vi "Teleop.vi"(10 "Match Info":T1={"Autonomous Elapsed Seconds"=0.0, "TeleOp Elapsed Seconds"=0.0, "Disabled Elapsed Seconds"=0.0, "Visited Autonomous"=FALSE, "Visited TeleOp"=FALSE, "Visited Disabled"=FALSE, "Autonomous Settings"={"Autonomous Style"=enum."Independent", "VI Refnum"=refnum}}, 11 "Call Context":T2) -> ()   [LabVIEW 2019]
doc: "This VI is called for each TeleOp packet received from the DS where the robot is not disabled. It is often used to read from the joysticks and update I/O or to update setpoints for timed control loops. It should complete and return within 20 milliseconds or it may miss DS packets."
uses:
  <vilib>/Rock Robotics/WPI/DriverStation/WPI_DriverStationDerivedRobotMode.ctl
  <vilib>/Rock Robotics/WPI/DriverStation/WPI_DriverStationMatch Info.ctl
  <vilib>/Rock Robotics/WPI/Utilities/WPI_GetSetVariantRefNum.vi
  <vilib>/Rock Robotics/Network Tables/NT Write Boolean Array.vi
  <vilib>/Rock Robotics/Network Tables/NT Write Numeric Array.vi
  <vilib>/Rock Robotics/Network Tables/NT Read Boolean.vi
  <vilib>/Rock Robotics/Network Tables/NT Write Boolean.vi
  <vilib>/Rock Robotics/Network Tables/NT Write Number.vi
  <vilib>/Rock Robotics/Network Tables/NT Read Number.vi
  <vilib>/Rock Robotics/Network Tables/NT Write String.vi
panel:
  out "Sample Slider 0":dbl(slide) scale=0.0..5.0
  out "Sample Boolean 1":bool
  out "Sample Boolean 0":bool
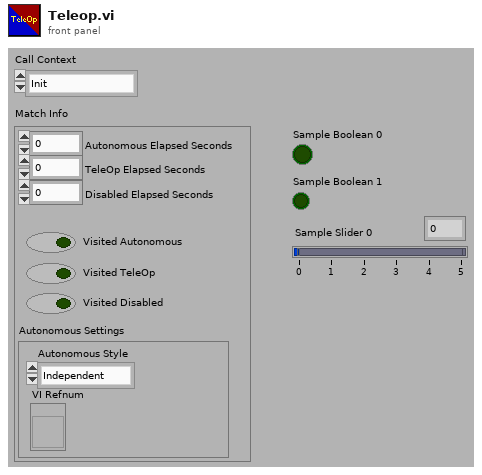
[diagram p1: front panel]
types:
  T1 = typedef "WPI_DriverStationMatch Info.ctl" = cluster{"Autonomous Elapsed Seconds":dbl, "TeleOp Elapsed Seconds":dbl, "Disabled Elapsed Seconds":dbl, "Visited Autonomous":bool, "Visited TeleOp":bool, "Visited Disabled":bool, "Autonomous Settings":cluster{"Autonomous Style":enum16{"Iterative", "Independent"}, "VI Refnum":refnum<vi>}}
  T2 = typedef "WPI_DriverStationDerivedRobotMode.ctl" = enum16{"Init", "Execute", "Stop"}
  T3 = typedef "WPI_JoystickDevRef.ctl" = cluster{"Device":T4}
  T4 = typedef "WPI_JoystickDeviceEnum.ctl" = enum16{"USB 0", "USB 1", "USB 2", "USB 3", "USB 4", "USB 5"}
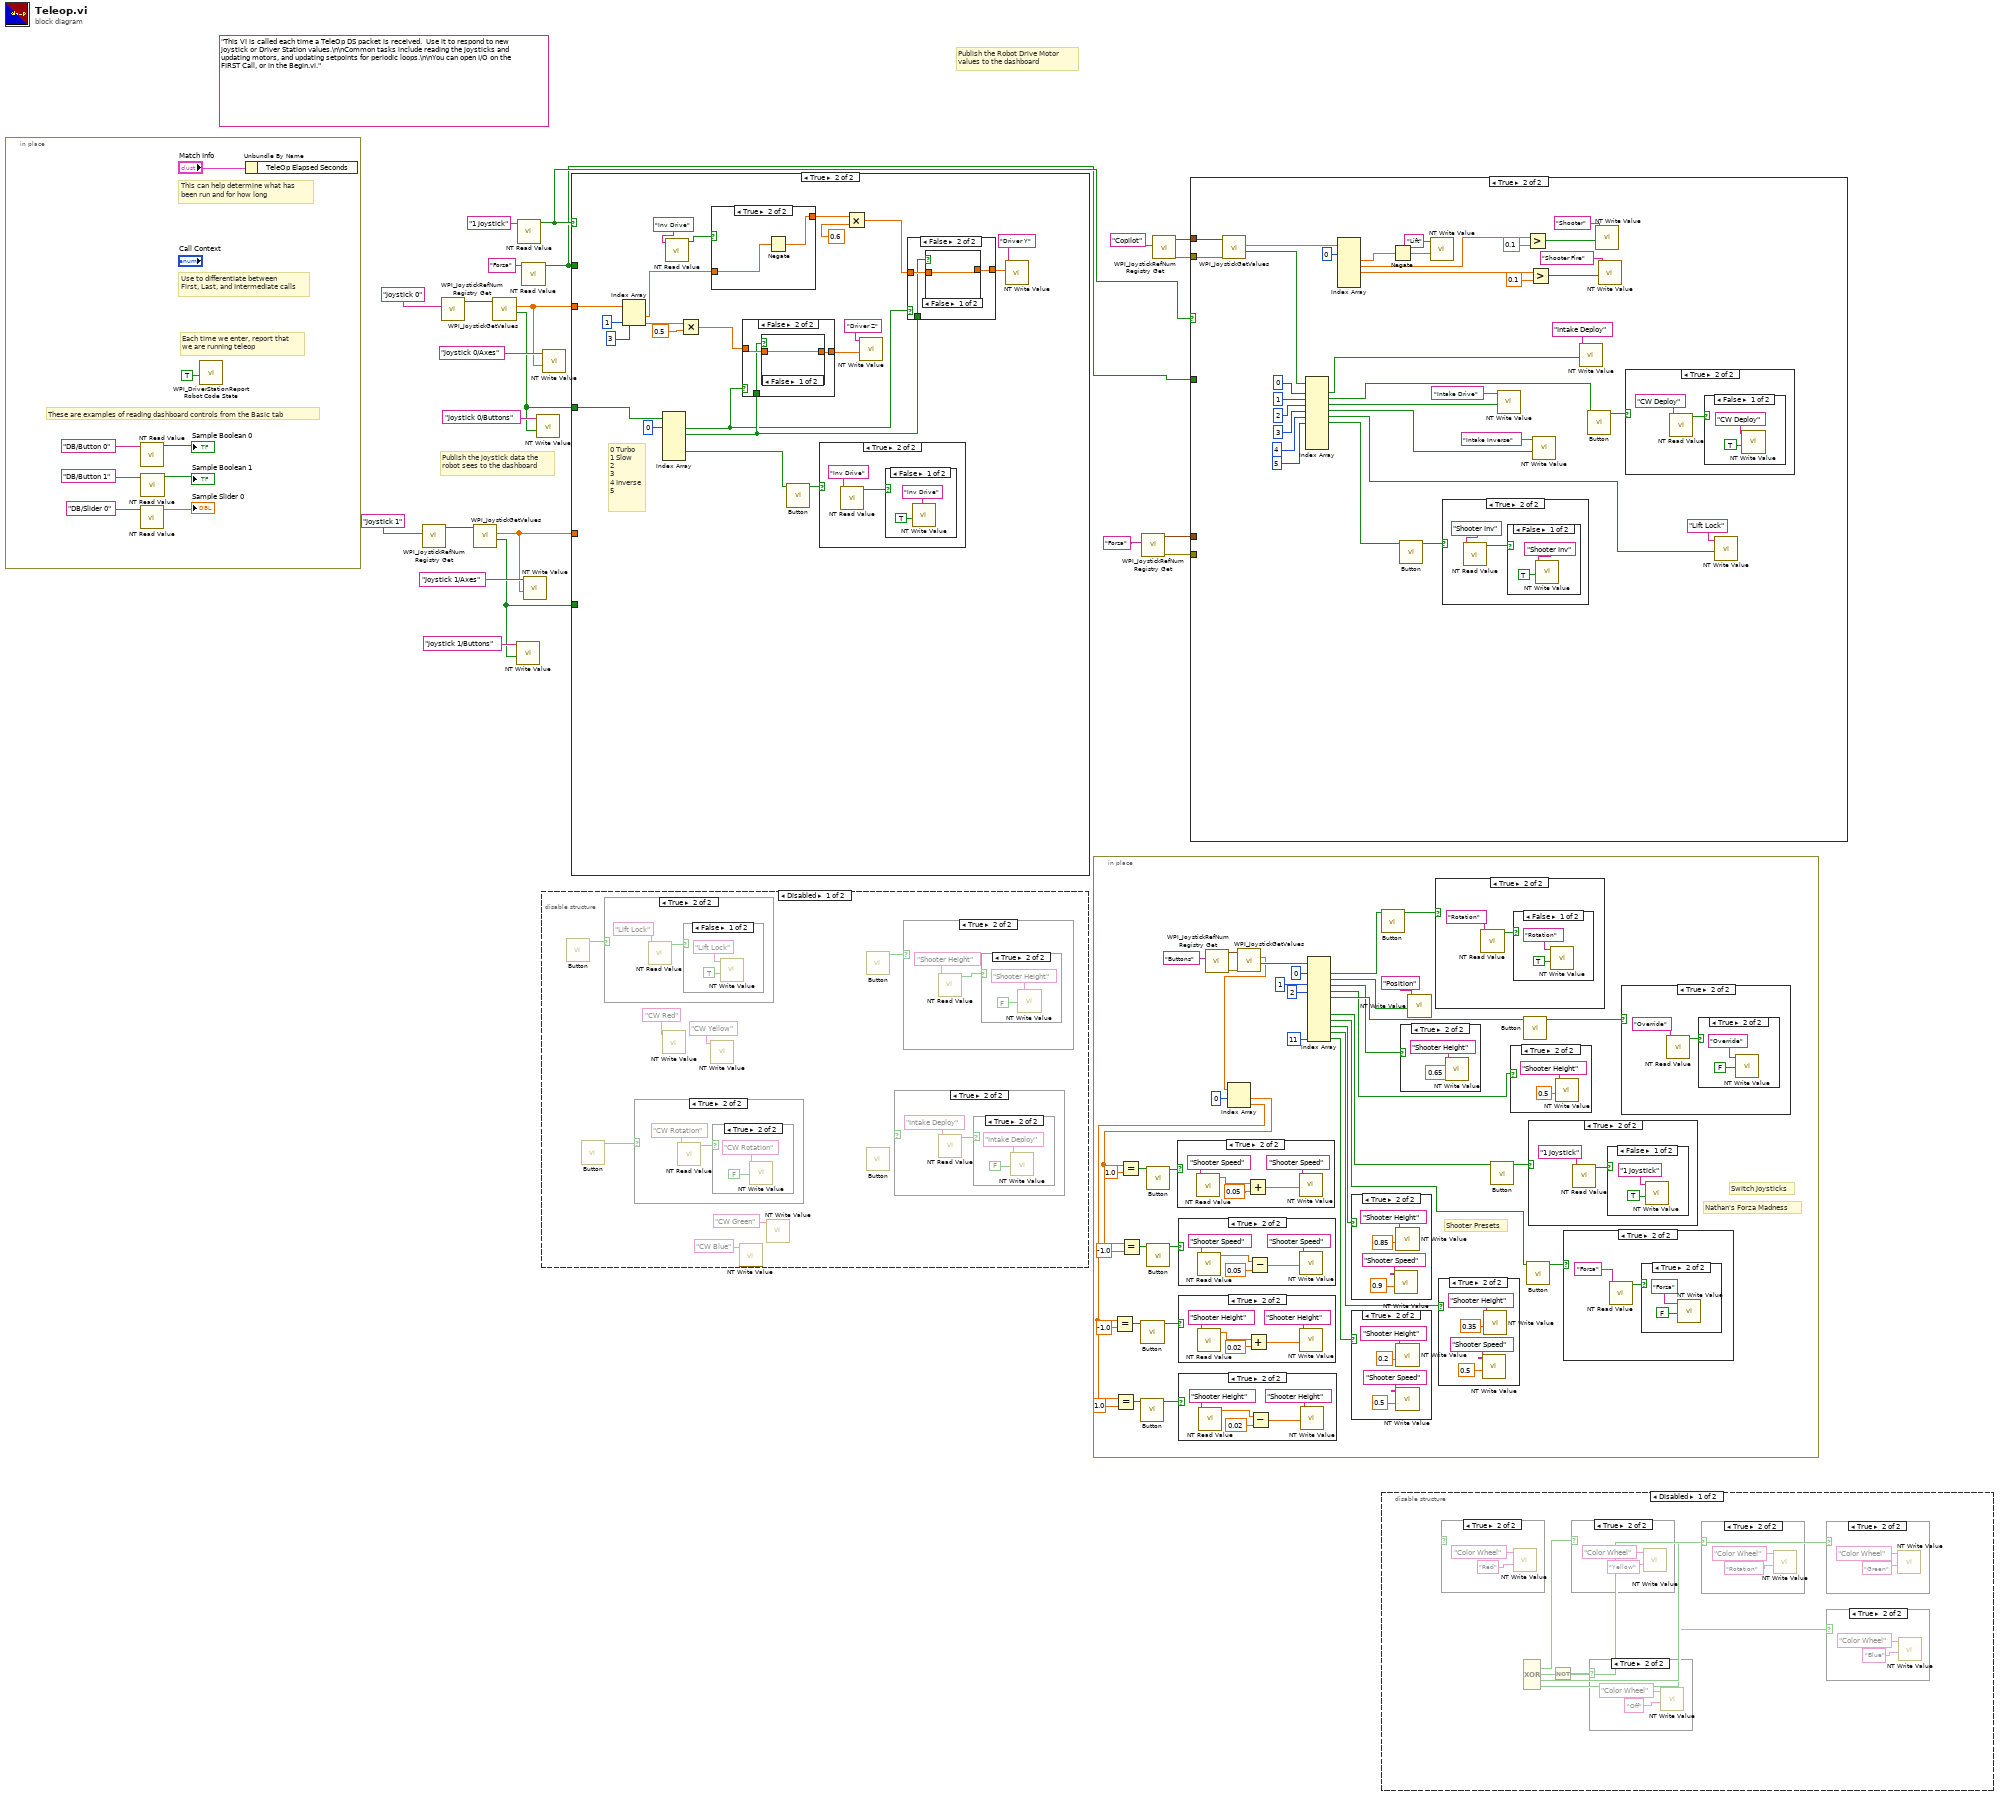
[diagram p0: block diagram]
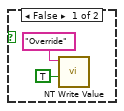
[diagram p9: hidden frame]
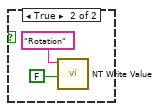
[diagram p11: hidden frame]
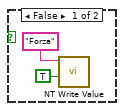
[diagram p14: hidden frame]
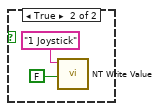
[diagram p16: hidden frame]
diagram:
  (unwired) "This VI is called each time a TeleOp DS packet is received.  Use it to respond to new joystick or Driver Station values.\n\nCommon tasks include reading the joysticks and updating motors, and updating setpoints for periodic loops.\n\nYou can open I/O on the FIRST Call, or in the Begin.vi."
  # "Publish the Robot Drive Motor\nvalues to the dashboard"
  # "Publish the joystick data the\nrobot sees to the dashboard"
  n1 = in-place {
    # "These are examples of reading dashboard controls from the Basic tab"
    # "Each time we enter, report that\nwe are running teleop"
    # "Use to differentiate between\nFirst, Last, and Intermediate calls"
    # "This can help determine what has\nbeen run and for how long"
    n2 = call-poly <vilib>:"NT Read Value.vi"("Name"="DB/Button 0" ("refnum name")) -> ("Boolean"=→"Sample Boolean 0":bool)  [unwired: 9 in, 1 out]
    n3 = call-poly <vilib>:"NT Read Value.vi"("Name"="DB/Slider 0" ("refnum name")) -> ("Numeric"=→"Sample Slider 0":dbl)  [unwired: 9 in, 1 out]
    n4 = call-poly <vilib>:"NT Read Value.vi"("Name"="DB/Button 1" ("refnum name")) -> ("Boolean"=→"Sample Boolean 1":bool)  [unwired: 9 in, 1 out]
    n5 = call <vilib>:"WPI_DriverStationReport Robot Code State.vi"("TeleOp"=TRUE ("Autonomous")) -> ()  [unwired: 10 in, 1 out]
    n6 = Unbundle By Name("Match Info") -> ()  [unwired: 1 out]
  }
  n7 = call <vilib>:"WPI_JoystickRefNum Registry Get.vi"("refnum name"="Joystick 1") -> ("JoystickDevRef"=w11:T3)  [unwired: 1 in, 9 out]
  n8 = call <vilib>:"WPI_JoystickRefNum Registry Get.vi"("refnum name"="Joystick 0") -> ("JoystickDevRef"=w21:T3)  [unwired: 1 in, 9 out]
  n9 = call <vilib>:"WPI_JoystickGetValues.vi"("JoystickDevRef"=w11) -> ("Buttons"=w7:bool[], "Axes"=w8:dbl[])  [unwired: 6 in, 3 out]
  n10 = call <vilib>:"WPI_JoystickGetValues.vi"("JoystickDevRef"=w21) -> ("Buttons"=w17:bool[], "Axes"=w18:dbl[])  [unwired: 6 in, 3 out]
  n11 = call-poly <vilib>:"NT Write Value.vi"("Boolean Array"=w7, "Name"="Joystick 1/Buttons") -> ()  [unwired: 9 in, 1 out]
  n12 = call-poly <vilib>:"NT Read Value.vi"("Name"="1 Joystick") -> ("Boolean"=w2:bool)  [unwired: 9 in, 1 out]
  n13 = call-poly <vilib>:"NT Read Value.vi"("Name"="Forza") -> ("Boolean"=w1:bool)  [unwired: 9 in, 1 out]
  n14 = call-poly <vilib>:"NT Write Value.vi"("Numeric Array"=w8, "Name"="Joystick 1/Axes") -> ()  [unwired: 9 in, 1 out]
  n15 = call-poly <vilib>:"NT Write Value.vi"("Boolean Array"=w17, "Name"="Joystick 0/Buttons") -> ()  [unwired: 9 in, 1 out]
  n16 = disable-structure shown="Disabled" {
    frame Disabled {
      n17 = call "Button.vi"() -> ("Button Pressed?"=w36:bool)  [unwired: 11 in]
      n18 = call "Button.vi"() -> ("Button Pressed?"=w31:bool)  [unwired: 11 in]
      n19 = case shown="True" w36 {
        frame False {
        }
        frame True {
          n20 = call-poly <vilib>:"NT Read Value.vi"("Name"="Lift Lock") -> ("Boolean"=w45:bool)  [unwired: 9 in, 1 out]
          n21 = case shown="False" w45 {
            frame False {
              n22 = call-poly <vilib>:"NT Write Value.vi"("Boolean"=TRUE, "Name"="Lift Lock") -> ()  [unwired: 9 in, 1 out]
            }
            frame True {
              n23 = call-poly <vilib>:"NT Write Value.vi"("Boolean"=FALSE, "Name"="Lift Lock") -> ()  [unwired: 9 in, 1 out]
            }
          }
        }
      }
      n24 = case shown="True" w31 {
        frame False {
        }
        frame True {
          n25 = call-poly <vilib>:"NT Read Value.vi"("Name"="CW Rotation") -> ("Boolean"=w39:bool)  [unwired: 9 in, 1 out]
          n26 = case shown="True" w39 {
            frame False {
              n27 = call-poly <vilib>:"NT Write Value.vi"("Boolean"=TRUE, "Name"="CW Rotation") -> ()  [unwired: 9 in, 1 out]
            }
            frame True {
              n28 = call-poly <vilib>:"NT Write Value.vi"("Boolean"=FALSE, "Name"="CW Rotation") -> ()  [unwired: 9 in, 1 out]
            }
          }
        }
      }
      n29 = call-poly <vilib>:"NT Write Value.vi"("Name"="CW Red") -> ()  [unwired: 10 in, 1 out]
      n30 = call-poly <vilib>:"NT Write Value.vi"("Name"="CW Yellow") -> ()  [unwired: 10 in, 1 out]
      n31 = call-poly <vilib>:"NT Write Value.vi"("Name"="CW Blue") -> ()  [unwired: 10 in, 1 out]
      n32 = call-poly <vilib>:"NT Write Value.vi"("Name"="CW Green") -> ()  [unwired: 10 in, 1 out]
      n33 = call "Button.vi"() -> ("Button Pressed?"=w38:bool)  [unwired: 11 in]
      n34 = call "Button.vi"() -> ()  [unwired: 11 in, 1 out]
      n35 = case shown="True" w37 {
        frame False {
        }
        frame True {
          n36 = call-poly <vilib>:"NT Read Value.vi"("Name"="Intake Deploy") -> ("Boolean"=w51:bool)  [unwired: 9 in, 1 out]
          n37 = case shown="True" w51 {
            frame False {
              n38 = call-poly <vilib>:"NT Write Value.vi"("Boolean"=TRUE, "Name"="Intake Deploy") -> ()  [unwired: 9 in, 1 out]
            }
            frame True {
              n39 = call-poly <vilib>:"NT Write Value.vi"("Boolean"=FALSE, "Name"="Intake Deploy") -> ()  [unwired: 9 in, 1 out]
            }
          }
        }
      }
      n40 = case shown="True" w38 {
        frame False {
        }
        frame True {
          n41 = call-poly <vilib>:"NT Read Value.vi"("Name"="Shooter Height") -> ("Boolean"=w57:bool)  [unwired: 9 in, 1 out]
          n42 = case shown="True" w57 {
            frame False {
              n43 = call-poly <vilib>:"NT Write Value.vi"("Boolean"=TRUE, "Name"="Shooter Height") -> ()  [unwired: 9 in, 1 out]
            }
            frame True {
              n44 = call-poly <vilib>:"NT Write Value.vi"("Boolean"=FALSE, "Name"="Shooter Height") -> ()  [unwired: 9 in, 1 out]
            }
          }
        }
      }
    }
    frame Enabled {
    }
  }
  n45 = call-poly <vilib>:"NT Write Value.vi"("Numeric Array"=w18, "Name"="Joystick 0/Axes") -> ()  [unwired: 9 in, 1 out]
  n46 = case shown="True" w2 {
    tunnel: w18 -> [w67 w175]
    tunnel: w17 -> [w66 w174]
    tunnel: w8 -> [w65 _]
    tunnel: w7 -> [w64 _]
    tunnel: w1 -> [w63 _]
    frame False {
      n47 = case shown="False" w63 {
        tunnel: w67 -> [_ w101]
        tunnel: w66 -> [_ w100]
        tunnel: w65 -> [_ w99]
        tunnel: w64 -> [_ w97]
        frame True {
        }
        frame False {
          # "0 Fire Shooter\n1 Intake Run\n2 Intake Inverse\n3 Lift Lock\n4 Turbo\n5 CW Deploy"
          # "0 Rev Shooter\n1 Intake Deploy\n2\n3\n4 Inverse\n5 Slow"
          n48 = Index Array(array=w101, index=1) -> (element=w106:dbl)
          n49 = call-poly <vilib>:"NT Read Value.vi"("Name"="Inv Drive") -> ("Boolean"=w80:bool)  [unwired: 9 in, 1 out]
          n50 = Index Array(array=w97, index #1=0 ("index")) -> (element #1=w88:bool, element #2=w85:bool, element #3=w73:bool, element #4=w74:bool, element #5=w79:bool, element #6=w82:bool)  [unwired: 5 in]
          n51 = Index Array(array=w100, index #1=0) -> (element #1=w84:bool, element #2=w70:bool, element #3=w68:bool, element #5=w77:bool, element #6=w76:bool)  [unwired: 5 in, 1 out]
          n52 = Index Array(array=w99, index=1) -> (element=w96:dbl)
          n53 = case shown="True" w80 {
            tunnel: w106 -> [w141 w143]
            tunnel: [w141 w142] -> w105
            frame False {
            }
            frame True {
              n54 = Negate(x=w143) -> (-x=w142:dbl)
            }
          }
          n55 = case shown="True" w80 {
            tunnel: w96 -> [w138 w140]
            tunnel: [w138 w139] -> w91
            frame False {
            }
            frame True {
              n56 = Negate(x=w140) -> (-x=w139:dbl)
            }
          }
          n57 = call-poly <vilib>:"NT Write Value.vi"("Boolean"=w88, "Name"="Shooter Fire") -> ()  [unwired: 9 in, 1 out]
          n58 = call-poly <vilib>:"NT Write Value.vi"("Boolean"=w84, "Name"="Shooter") -> ()  [unwired: 9 in, 1 out]
          n59 = call-poly <vilib>:"NT Write Value.vi"("Boolean"=w85, "Name"="Intake Drive") -> ()  [unwired: 9 in, 1 out]
          n60 = call "Button.vi"("Button In"=w74) -> ("Button Pressed?"=w75:bool)  [unwired: 10 in]
          n61 = call-poly <vilib>:"NT Write Value.vi"("Boolean"=w73, "Name"="Intake Inverse") -> ()  [unwired: 9 in, 1 out]
          n62 = Multiply(x=w105, y=0.75) -> (x*y=w104:dbl)
          n63 = call-poly <vilib>:"NT Write Value.vi"("Boolean"=w70, "Name"="Intake Deploy") -> ()  [unwired: 9 in, 1 out]
          n64 = Multiply(x=w91, y=0.75) -> (x*y=w94:dbl)
          n65 = call "Button.vi"("Button In"=w82) -> ("Button Pressed?"=w83:bool)  [unwired: 10 in]
          n66 = call "Button.vi"("Button In"=w77) -> ("Button Pressed?"=w78:bool)  [unwired: 10 in]
          n67 = case shown="True" w75 {
            frame False {
            }
            frame True {
              n68 = call-poly <vilib>:"NT Read Value.vi"("Name"="Lift Lock") -> ("Boolean"=w110:bool)  [unwired: 9 in, 1 out]
              n69 = case shown="False" w110 {
                frame False {
                  n70 = call-poly <vilib>:"NT Write Value.vi"("Boolean"=TRUE, "Name"="Lift Lock") -> ()  [unwired: 9 in, 1 out]
                }
                frame True {
                  n71 = call-poly <vilib>:"NT Write Value.vi"("Boolean"=FALSE, "Name"="Lift Lock") -> ()  [unwired: 9 in, 1 out]
                }
              }
            }
          }
          n72 = case shown="True" w83 {
            frame False {
            }
            frame True {
              n73 = call-poly <vilib>:"NT Read Value.vi"("Name"="CW Deploy") -> ("Boolean"=w122:bool)  [unwired: 9 in, 1 out]
              n74 = case shown="False" w122 {
                frame False {
                  n75 = call-poly <vilib>:"NT Write Value.vi"("Boolean"=TRUE, "Name"="CW Deploy") -> ()  [unwired: 9 in, 1 out]
                }
                frame True {
                  n76 = call-poly <vilib>:"NT Write Value.vi"("Boolean"=FALSE, "Name"="CW Deploy") -> ()  [unwired: 9 in, 1 out]
                }
              }
            }
          }
          n77 = case shown="False" w79 {
            tunnel: w104 -> [w145 w149]
            tunnel: [w144 w148] -> w103
            tunnel: w76 -> [_ w147]
            frame True {
              n78 = Multiply(x=w145, y=1.33) -> (x*y=w144:dbl)
            }
            frame False {
              n79 = case shown="True" w147 {
                tunnel: w149 -> [w150 w152]
                tunnel: [w150 w151] -> w148
                frame False {
                }
                frame True {
                  n80 = Multiply(x=w152, y=0.66) -> (x*y=w151:dbl)
                }
              }
            }
          }
          n81 = case shown="False" w79 {
            tunnel: w94 -> [w129 w133]
            tunnel: [w128 w132] -> w93
            tunnel: w76 -> [_ w131]
            frame True {
              n82 = Multiply(x=w129, y=1.33) -> (x*y=w128:dbl)
            }
            frame False {
              n83 = case shown="True" w131 {
                tunnel: w133 -> [w134 w136]
                tunnel: [w134 w135] -> w132
                frame False {
                }
                frame True {
                  n84 = Multiply(x=w136, y=0.66) -> (x*y=w135:dbl)
                }
              }
            }
          }
          n85 = case shown="True" w78 {
            frame False {
            }
            frame True {
              n86 = call-poly <vilib>:"NT Read Value.vi"("Name"="Inv Drive") -> ("Boolean"=w116:bool)  [unwired: 9 in, 1 out]
              n87 = case shown="False" w116 {
                frame False {
                  n88 = call-poly <vilib>:"NT Write Value.vi"("Boolean"=TRUE, "Name"="Inv Drive") -> ()  [unwired: 9 in, 1 out]
                }
                frame True {
                  n89 = call-poly <vilib>:"NT Write Value.vi"("Boolean"=FALSE, "Name"="Inv Drive") -> ()  [unwired: 9 in, 1 out]
                }
              }
            }
          }
          n90 = call-poly <vilib>:"NT Write Value.vi"("Boolean"=w68, "Name"="Shooter Nerf") -> ()  [unwired: 9 in, 1 out]
          n91 = call-poly <vilib>:"NT Write Value.vi"("Numeric"=w103, "Name"="Driver Y") -> ()  [unwired: 9 in, 1 out]
          n92 = call-poly <vilib>:"NT Write Value.vi"("Numeric"=w93, "Name"="Driver Z") -> ()  [unwired: 9 in, 1 out]
        }
      }
    }
    frame True {
      # "0 Turbo\n1 Slow\n2\n3\n4 Inverse\n5"
      n93 = Index Array(array=w175, index #1=1, index #2=3) -> (element #1=w169:dbl, element #2=w164:dbl)
      n94 = Index Array(array=w174, index #1=0) -> (element #1=w158:bool, element #2=w159:bool, element #5=w156:bool)  [unwired: 5 in, 3 out]
      n95 = call-poly <vilib>:"NT Read Value.vi"("Name"="Inv Drive") -> ("Boolean"=w155:bool)  [unwired: 9 in, 1 out]
      n96 = Multiply(x=w164, y=0.5) -> (x*y=w165:dbl)
      n97 = case shown="True" w155 {
        tunnel: w169 -> [w192 w194]
        tunnel: [w192 w193] -> w168
        frame False {
        }
        frame True {
          n98 = Negate(x=w194) -> (-x=w193:dbl)
        }
      }
      n99 = case shown="False" w158 {
        tunnel: [w182 w186] -> w163
        tunnel: w165 -> [w183 w187]
        tunnel: w159 -> [_ w185]
        frame True {
          n100 = Multiply(x=w183, y=1.33) -> (x*y=w182:dbl)
        }
        frame False {
          n101 = case shown="False" w185 {
            tunnel: [w188 w190] -> w186
            tunnel: w187 -> [w188 w189]
            frame False {
            }
            frame True {
              n102 = Multiply(x=w189, y=0.66) -> (x*y=w190:dbl)
            }
          }
        }
      }
      n103 = call "Button.vi"("Button In"=w156) -> ("Button Pressed?"=w157:bool)  [unwired: 10 in]
      n104 = case shown="True" w157 {
        frame False {
        }
        frame True {
          n105 = call-poly <vilib>:"NT Read Value.vi"("Name"="Inv Drive") -> ("Boolean"=w176:bool)  [unwired: 9 in, 1 out]
          n106 = case shown="False" w176 {
            frame False {
              n107 = call-poly <vilib>:"NT Write Value.vi"("Boolean"=TRUE, "Name"="Inv Drive") -> ()  [unwired: 9 in, 1 out]
            }
            frame True {
              n108 = call-poly <vilib>:"NT Write Value.vi"("Boolean"=FALSE, "Name"="Inv Drive") -> ()  [unwired: 9 in, 1 out]
            }
          }
        }
      }
      n109 = Multiply(x=w168, y=0.6) -> (x*y=w167:dbl)
      n110 = call-poly <vilib>:"NT Write Value.vi"("Numeric"=w163, "Name"="Driver Z") -> ()  [unwired: 9 in, 1 out]
      n111 = case shown="False" w158 {
        tunnel: w167 -> [w196 w200]
        tunnel: [w195 w199] -> w161
        tunnel: w159 -> [_ w198]
        frame True {
          n112 = Multiply(x=w196, y=1.33) -> (x*y=w195:dbl)
        }
        frame False {
          n113 = case shown="False" w198 {
            tunnel: w200 -> [w201 w203]
            tunnel: [w201 w202] -> w199
            frame False {
            }
            frame True {
              n114 = Multiply(x=w203, y=0.66) -> (x*y=w202:dbl)
            }
          }
        }
      }
      n115 = call-poly <vilib>:"NT Write Value.vi"("Numeric"=w161, "Name"="Driver Y") -> ()  [unwired: 9 in, 1 out]
    }
  }
  n116 = in-place {
    # "Shooter Presets"
    # "Nathan's Forza Madness"
    # "Switch Joysticks"
    n117 = call <vilib>:"WPI_JoystickRefNum Registry Get.vi"("refnum name"="Buttons") -> ("error out"=w243:errorcluster, "JoystickDevRef"=w242:T3)  [unwired: 9 in]
    n118 = call <vilib>:"WPI_JoystickGetValues.vi"("error in (no error)"=w243, "JoystickDevRef"=w242) -> ("Buttons"=w240:bool[], "Axes"=w220:dbl[])  [unwired: 5 in, 3 out]
    n119 = Index Array(array=w220, index #1=0 ("index")) -> (element #1=w218:dbl, element #2=w213:dbl)  [unwired: 1 in]
    n120 = Equal?(x=w213, y=-1.0) -> (x = y?=w210:bool)
    n121 = Equal?(x=w213, y=1.0) -> (x = y?=w211:bool)
    n122 = Equal?(x=w218, y=1.0) -> (x = y?=w206:bool)
    n123 = Equal?(x=w218, y=-1.0) -> (x = y?=w208:bool)
    n124 = call "Button.vi"("Button In"=w211) -> ("Button Pressed?"=w212:bool)  [unwired: 10 in]
    n125 = call "Button.vi"("Button In"=w210) -> ("Button Pressed?"=w209:bool)  [unwired: 10 in]
    n126 = call "Button.vi"("Button In"=w206) -> ("Button Pressed?"=w205:bool)  [unwired: 10 in]
    n127 = call "Button.vi"("Button In"=w208) -> ("Button Pressed?"=w207:bool)  [unwired: 10 in]
    n128 = case shown="True" w205 {
      frame False {
      }
      frame True {
        n129 = call-poly <vilib>:"NT Read Value.vi"("Name"="Shooter Speed") -> ("Numeric"=w261:dbl)  [unwired: 9 in, 1 out]
        n130 = Add(x=w261, y=0.05) -> (x+y=w260:dbl)
        n131 = call-poly <vilib>:"NT Write Value.vi"("Numeric"=w260, "Name"="Shooter Speed") -> ()  [unwired: 9 in, 1 out]
      }
    }
    n132 = case shown="True" w207 {
      frame False {
      }
      frame True {
        n133 = call-poly <vilib>:"NT Read Value.vi"("Name"="Shooter Speed") -> ("Numeric"=w255:dbl)  [unwired: 9 in, 1 out]
        n134 = Subtract(x=w255, y=0.05) -> (x-y=w256:dbl)
        n135 = call-poly <vilib>:"NT Write Value.vi"("Numeric"=w256, "Name"="Shooter Speed") -> ()  [unwired: 9 in, 1 out]
      }
    }
    n136 = case shown="True" w209 {
      frame False {
      }
      frame True {
        n137 = call-poly <vilib>:"NT Read Value.vi"("Name"="Shooter Height") -> ("Numeric"=w251:dbl)  [unwired: 9 in, 1 out]
        n138 = Add(x=w251, y=0.02) -> (x+y=w250:dbl)
        n139 = call-poly <vilib>:"NT Write Value.vi"("Numeric"=w250, "Name"="Shooter Height") -> ()  [unwired: 9 in, 1 out]
      }
    }
    n140 = case shown="True" w212 {
      frame False {
      }
      frame True {
        n141 = call-poly <vilib>:"NT Read Value.vi"("Name"="Shooter Height") -> ("Numeric"=w245:dbl)  [unwired: 9 in, 1 out]
        n142 = Subtract(x=w245, y=0.02) -> (x-y=w246:dbl)
        n143 = call-poly <vilib>:"NT Write Value.vi"("Numeric"=w246, "Name"="Shooter Height") -> ()  [unwired: 9 in, 1 out]
      }
    }
    n144 = Index Array(array=w240, index #1=0 ("index"), index #2=1 ("index"), index #3=2 ("index"), index #12=11 ("index")) -> (element #1=w226:bool, element #2=w224:bool, element #3=w222:bool, element #4=w221:bool, element #5=w223:bool, element #8=w235:bool, element #9=w233:bool, element #10=w237:bool, element #11=w238:bool, element #12=w229:bool)  [unwired: 8 in, 2 out]
    n145 = case shown="True" w237 {
      frame False {
      }
      frame True {
        n146 = call-poly <vilib>:"NT Write Value.vi"("Numeric"=0.9, "Name"="Shooter Speed") -> ()  [unwired: 9 in, 1 out]
        n147 = call-poly <vilib>:"NT Write Value.vi"("Numeric"=0.85, "Name"="Shooter Height") -> ()  [unwired: 9 in, 1 out]
      }
    }
    n148 = case shown="True" w229 {
      frame False {
      }
      frame True {
        n149 = call-poly <vilib>:"NT Write Value.vi"("Numeric"=0.2, "Name"="Shooter Height") -> ()  [unwired: 9 in, 1 out]
        n150 = call-poly <vilib>:"NT Write Value.vi"("Numeric"=0.5, "Name"="Shooter Speed") -> ()  [unwired: 9 in, 1 out]
      }
    }
    n151 = call "Button.vi"("Button In"=w226) -> ("Button Pressed?"=w228:bool)  [unwired: 10 in]
    n152 = case shown="True" w222 {
      frame False {
      }
      frame True {
        n153 = call-poly <vilib>:"NT Write Value.vi"("Numeric"=0.65, "Name"="Shooter Height") -> ()  [unwired: 9 in, 1 out]
      }
    }
    n154 = call-poly <vilib>:"NT Write Value.vi"("Boolean"=w224, "Name"="Position") -> ()  [unwired: 9 in, 1 out]
    n155 = case shown="True" w228 {
      frame False {
      }
      frame True {
        n156 = call-poly <vilib>:"NT Read Value.vi"("Name"="Rotation") -> ("Boolean"=w274:bool)  [unwired: 9 in, 1 out]
        n157 = case shown="False" w274 {
          frame False {
            n158 = call-poly <vilib>:"NT Write Value.vi"("Boolean"=TRUE, "Name"="Rotation") -> ()  [unwired: 9 in, 1 out]
          }
          frame True {
            n159 = call-poly <vilib>:"NT Write Value.vi"("Boolean"=FALSE, "Name"="Rotation") -> ()  [unwired: 9 in, 1 out]
          }
        }
      }
    }
    n160 = case shown="True" w238 {
      frame False {
      }
      frame True {
        n161 = call-poly <vilib>:"NT Write Value.vi"("Numeric"=0.5, "Name"="Shooter Speed") -> ()  [unwired: 9 in, 1 out]
        n162 = call-poly <vilib>:"NT Write Value.vi"("Numeric"=0.35, "Name"="Shooter Height") -> ()  [unwired: 9 in, 1 out]
      }
    }
    n163 = call "Button.vi"("Button In"=w235) -> ("Button Pressed?"=w236:bool)  [unwired: 10 in]
    n164 = case shown="True" w221 {
      frame False {
      }
      frame True {
        n165 = call-poly <vilib>:"NT Write Value.vi"("Numeric"=0.5, "Name"="Shooter Height") -> ()  [unwired: 9 in, 1 out]
      }
    }
    n166 = call "Button.vi"("Button In"=w223) -> ("Button Pressed?"=w227:bool)  [unwired: 10 in]
    n167 = call "Button.vi"("Button In"=w233) -> ("Button Pressed?"=w234:bool)  [unwired: 10 in]
    n168 = case shown="True" w236 {
      frame False {
      }
      frame True {
        n169 = call-poly <vilib>:"NT Read Value.vi"("Name"="1 Joystick") -> ("Boolean"=w290:bool)  [unwired: 9 in, 1 out]
        n170 = case shown="False" w290 {
          frame False {
            n171 = call-poly <vilib>:"NT Write Value.vi"("Boolean"=TRUE, "Name"="1 Joystick") -> ()  [unwired: 9 in, 1 out]
          }
          frame True {
            n172 = call-poly <vilib>:"NT Write Value.vi"("Boolean"=FALSE, "Name"="1 Joystick") -> ()  [unwired: 9 in, 1 out]
          }
        }
      }
    }
    n173 = case shown="True" w234 {
      frame False {
      }
      frame True {
        n174 = call-poly <vilib>:"NT Read Value.vi"("Name"="Forza") -> ("Boolean"=w284:bool)  [unwired: 9 in, 1 out]
        n175 = case shown="True" w284 {
          frame False {
            n176 = call-poly <vilib>:"NT Write Value.vi"("Boolean"=TRUE, "Name"="Forza") -> ()  [unwired: 9 in, 1 out]
          }
          frame True {
            n177 = call-poly <vilib>:"NT Write Value.vi"("Boolean"=FALSE, "Name"="Forza") -> ()  [unwired: 9 in, 1 out]
          }
        }
      }
    }
    n178 = case shown="True" w227 {
      frame False {
      }
      frame True {
        n179 = call-poly <vilib>:"NT Read Value.vi"("Name"="Override") -> ("Boolean"=w268:bool)  [unwired: 9 in, 1 out]
        n180 = case shown="True" w268 {
          frame False {
            n181 = call-poly <vilib>:"NT Write Value.vi"("Boolean"=TRUE, "Name"="Override") -> ()  [unwired: 9 in, 1 out]
          }
          frame True {
            n182 = call-poly <vilib>:"NT Write Value.vi"("Boolean"=FALSE, "Name"="Override") -> ()  [unwired: 9 in, 1 out]
          }
        }
      }
    }
  }
  n183 = call <vilib>:"WPI_JoystickRefNum Registry Get.vi"("refnum name"="Forza") -> ("error out"=w3:errorcluster, "JoystickDevRef"=w4:T3)  [unwired: 9 in]
  n184 = call <vilib>:"WPI_JoystickRefNum Registry Get.vi"("refnum name"="Copilot") -> ("error out"=w16:errorcluster, "JoystickDevRef"=w15:T3)  [unwired: 9 in]
  n185 = case shown="True" w2 {
    tunnel: w16 -> [w307 w457]
    tunnel: w15 -> [w308 w456]
    tunnel: w1 -> [w306 _]
    tunnel: w4 -> [w305 _]
    tunnel: w3 -> [w304 _]
    frame False {
      n186 = case shown="True" w306 {
        tunnel: w308 -> [_ w368]
        tunnel: w307 -> [_ w367]
        tunnel: w305 -> [_ w361]
        tunnel: w304 -> [_ w360]
        frame False {
        }
        frame True {
          n187 = call <vilib>:"WPI_JoystickGetValues.vi"("error in (no error)"=w360, "JoystickDevRef"=w361) -> ("Buttons"=w365:bool[], "Axes"=w366:dbl[])  [unwired: 5 in, 3 out]
          n188 = call <vilib>:"WPI_JoystickGetValues.vi"("error in (no error)"=w367, "JoystickDevRef"=w368) -> ("Buttons"=w337:bool[], "Axes"=w338:dbl[])  [unwired: 5 in, 3 out]
          n189 = Index Array(array=w337, index #1=0, index #2=1, index #3=2, index #4=3) -> (element #1=w320:bool, element #2=w347:bool, element #3=w348:bool, element #4=w323:bool, element #5=w322:bool, element #6=w311:bool)  [unwired: 6 in, 4 out]
          n190 = Index Array(array=w338, index #1=0 ("index")) -> (element #2=w343:dbl, element #3=w353:dbl, element #4=w339:dbl)  [unwired: 5 in, 3 out]
          n191 = Index Array(array=w365, index #1=0 ("index")) -> (element #1=w317:bool, element #2=w318:bool, element #5=w315:bool)  [unwired: 9 in, 7 out]
          n192 = Index Array(array=w366, index #1=0 ("index")) -> (element #1=w327:dbl, element #3=w363:dbl, element #4=w336:dbl)  [unwired: 5 in, 3 out]
          n193 = Negate(x=w343) -> (-x=w344:dbl)
          n194 = call-poly <vilib>:"NT Write Value.vi"("Numeric"=w344, "Name"="Lift") -> ()  [unwired: 9 in, 1 out]
          n195 = Negate(x=w363) -> (-x=w362:dbl)
          n196 = Add(x=w362, y=w336) -> (x+y=w328:dbl)
          n197 = call-poly <vilib>:"NT Read Value.vi"("Name"="Override") -> ("Boolean"=w309:bool)  [unwired: 9 in, 1 out]
          n198 = Multiply(x=0.7, y=w327) -> (x*y=w333:dbl)
          n199 = case shown="False" w309 {
            tunnel: w333 -> [w370 w375]
            tunnel: [w369 w374] -> w332
            tunnel: w318 -> [_ w373]
            tunnel: w317 -> [_ w372]
            frame True {
              n200 = Multiply(x=w370, y=0.3) -> (x*y=w369:dbl)
            }
            frame False {
              n201 = case shown="False" w372 {
                tunnel: [w376 w380] -> w374
                tunnel: w375 -> [w377 w381]
                tunnel: w373 -> [_ w379]
                frame True {
                  n202 = Multiply(x=w377, y=0.5) -> (x*y=w376:dbl)
                }
                frame False {
                  n203 = case shown="False" w379 {
                    tunnel: [w382 w384] -> w380
                    tunnel: w381 -> [w382 w383]
                    frame False {
                    }
                    frame True {
                      n204 = Multiply(x=w383, y=1.33) -> (x*y=w384:dbl)
                    }
                  }
                }
              }
            }
          }
          n205 = call-poly <vilib>:"NT Read Value.vi"("Name"="Inv Drive") -> ("Boolean"=w313:bool)  [unwired: 9 in, 1 out]
          n206 = call-poly <vilib>:"NT Write Value.vi"("Boolean"=w348, "Name"="Intake Drive") -> ()  [unwired: 9 in, 1 out]
          n207 = Greater?(x=w353, y=0.1) -> (0:w350:bool)
          n208 = Greater?(x=w339, y=0.1) -> (0:w340:bool)
          n209 = case shown="True" w313 {
            tunnel: [w415 w417] -> w335
            tunnel: w328 -> [w415 w416]
            frame False {
            }
            frame True {
              n210 = Negate(x=w416) -> (-x=w417:dbl)
            }
          }
          n211 = call-poly <vilib>:"NT Write Value.vi"("Boolean"=w322, "Name"="Lift Lock") -> ()  [unwired: 9 in, 1 out]
          n212 = call-poly <vilib>:"NT Write Value.vi"("Boolean"=w350, "Name"="Shooter") -> ()  [unwired: 9 in, 1 out]
          n213 = call-poly <vilib>:"NT Write Value.vi"("Boolean"=w340, "Name"="Shooter Fire") -> ()  [unwired: 9 in, 1 out]
          n214 = call-poly <vilib>:"NT Write Value.vi"("Boolean"=w320, "Name"="Intake Deploy") -> ()  [unwired: 9 in, 1 out]
          n215 = call "Button.vi"("Button In"=w347) -> ("Button Pressed?"=w346:bool)  [unwired: 10 in]
          n216 = call-poly <vilib>:"NT Write Value.vi"("Boolean"=w323, "Name"="Intake Inverse") -> ()  [unwired: 9 in, 1 out]
          n217 = call-poly <vilib>:"NT Write Value.vi"("Numeric"=w332, "Name"="Driver Z") -> ()  [unwired: 9 in, 1 out]
          n218 = call "Button.vi"("Button In"=w311) -> ("Button Pressed?"=w312:bool)  [unwired: 10 in]
          n219 = Multiply(x=w335, y=0.6) -> (x*y=w334:dbl)
          n220 = call "Button.vi"("Button In"=w315) -> ("Button Pressed?"=w316:bool)  [unwired: 10 in]
          n221 = case shown="True" w346 {
            frame False {
            }
            frame True {
              n222 = call-poly <vilib>:"NT Read Value.vi"("Name"="CW Deploy") -> ("Boolean"=w418:bool)  [unwired: 9 in, 1 out]
              n223 = case shown="False" w418 {
                frame False {
                  n224 = call-poly <vilib>:"NT Write Value.vi"("Boolean"=TRUE, "Name"="CW Deploy") -> ()  [unwired: 9 in, 1 out]
                }
                frame True {
                  n225 = call-poly <vilib>:"NT Write Value.vi"("Boolean"=FALSE, "Name"="CW Deploy") -> ()  [unwired: 9 in, 1 out]
                }
              }
            }
          }
          n226 = case shown="True" w312 {
            frame False {
            }
            frame True {
              n227 = call-poly <vilib>:"NT Read Value.vi"("Name"="Shooter Inv") -> ("Boolean"=w403:bool)  [unwired: 9 in, 1 out]
              n228 = case shown="False" w403 {
                frame False {
                  n229 = call-poly <vilib>:"NT Write Value.vi"("Boolean"=TRUE, "Name"="Shooter Inv") -> ()  [unwired: 9 in, 1 out]
                }
                frame True {
                  n230 = call-poly <vilib>:"NT Write Value.vi"("Boolean"=FALSE, "Name"="Shooter Inv") -> ()  [unwired: 9 in, 1 out]
                }
              }
            }
          }
          n231 = case shown="False" w309 {
            tunnel: w334 -> [w386 w392]
            tunnel: [w387 w391] -> w330
            tunnel: w318 -> [_ w390]
            tunnel: w317 -> [_ w389]
            frame True {
              n232 = Multiply(x=w386, y=0.3) -> (x*y=w387:dbl)
            }
            frame False {
              n233 = case shown="False" w389 {
                tunnel: w392 -> [w394 w398]
                tunnel: [w393 w397] -> w391
                tunnel: w390 -> [_ w396]
                frame True {
                  n234 = Multiply(x=w394, y=0.5) -> (x*y=w393:dbl)
                }
                frame False {
                  n235 = case shown="False" w396 {
                    tunnel: w398 -> [w399 w401]
                    tunnel: [w399 w400] -> w397
                    frame False {
                    }
                    frame True {
                      n236 = Multiply(x=w401, y=1.33) -> (x*y=w400:dbl)
                    }
                  }
                }
              }
            }
          }
          n237 = case shown="True" w316 {
            frame False {
            }
            frame True {
              n238 = call-poly <vilib>:"NT Read Value.vi"("Name"="Inv Drive") -> ("Boolean"=w409:bool)  [unwired: 9 in, 1 out]
              n239 = case shown="False" w409 {
                frame False {
                  n240 = call-poly <vilib>:"NT Write Value.vi"("Boolean"=TRUE, "Name"="Inv Drive") -> ()  [unwired: 9 in, 1 out]
                }
                frame True {
                  n241 = call-poly <vilib>:"NT Write Value.vi"("Boolean"=FALSE, "Name"="Inv Drive") -> ()  [unwired: 9 in, 1 out]
                }
              }
            }
          }
          n242 = call-poly <vilib>:"NT Write Value.vi"("Numeric"=w330, "Name"="Driver Y") -> ()  [unwired: 9 in, 1 out]
        }
      }
    }
    frame True {
      n243 = call <vilib>:"WPI_JoystickGetValues.vi"("error in (no error)"=w457, "JoystickDevRef"=w456) -> ("Buttons"=w454:bool[], "Axes"=w455:dbl[])  [unwired: 5 in, 3 out]
      n244 = Index Array(array=w454, index #1=0, index #2=1, index #3=2, index #4=3, index #5=4 ("index"), index #6=5 ("index")) -> (element #1=w428:bool, element #2=w442:bool, element #3=w443:bool, element #4=w432:bool, element #5=w427:bool, element #6=w424:bool)  [unwired: 4 in, 4 out]
      n245 = Index Array(array=w455, index #1=0 ("index")) -> (element #2=w438:dbl, element #3=w448:dbl, element #4=w434:dbl)  [unwired: 5 in, 3 out]
      n246 = Negate(x=w438) -> (-x=w439:dbl)
      n247 = call "Button.vi"("Button In"=w424) -> ("Button Pressed?"=w425:bool)  [unwired: 10 in]
      n248 = call-poly <vilib>:"NT Write Value.vi"("Numeric"=w439, "Name"="Lift") -> ()  [unwired: 9 in, 1 out]
      n249 = case shown="True" w425 {
        frame False {
        }
        frame True {
          n250 = call-poly <vilib>:"NT Read Value.vi"("Name"="Shooter Inv") -> ("Boolean"=w458:bool)  [unwired: 9 in, 1 out]
          n251 = case shown="False" w458 {
            frame False {
              n252 = call-poly <vilib>:"NT Write Value.vi"("Boolean"=TRUE, "Name"="Shooter Inv") -> ()  [unwired: 9 in, 1 out]
            }
            frame True {
              n253 = call-poly <vilib>:"NT Write Value.vi"("Boolean"=FALSE, "Name"="Shooter Inv") -> ()  [unwired: 9 in, 1 out]
            }
          }
        }
      }
      n254 = call-poly <vilib>:"NT Write Value.vi"("Boolean"=w443, "Name"="Intake Drive") -> ()  [unwired: 9 in, 1 out]
      n255 = Greater?(x=w448, y=0.1) -> (0:w445:bool)
      n256 = Greater?(x=w434, y=0.1) -> (0:w435:bool)
      n257 = call-poly <vilib>:"NT Write Value.vi"("Boolean"=w432, "Name"="Intake Inverse") -> ()  [unwired: 9 in, 1 out]
      n258 = call-poly <vilib>:"NT Write Value.vi"("Boolean"=w428, "Name"="Intake Deploy") -> ()  [unwired: 9 in, 1 out]
      n259 = call "Button.vi"("Button In"=w442) -> ("Button Pressed?"=w441:bool)  [unwired: 10 in]
      n260 = call-poly <vilib>:"NT Write Value.vi"("Boolean"=w445, "Name"="Shooter") -> ()  [unwired: 9 in, 1 out]
      n261 = call-poly <vilib>:"NT Write Value.vi"("Boolean"=w435, "Name"="Shooter Fire") -> ()  [unwired: 9 in, 1 out]
      n262 = case shown="True" w441 {
        frame False {
        }
        frame True {
          n263 = call-poly <vilib>:"NT Read Value.vi"("Name"="CW Deploy") -> ("Boolean"=w464:bool)  [unwired: 9 in, 1 out]
          n264 = case shown="False" w464 {
            frame False {
              n265 = call-poly <vilib>:"NT Write Value.vi"("Boolean"=TRUE, "Name"="CW Deploy") -> ()  [unwired: 9 in, 1 out]
            }
            frame True {
              n266 = call-poly <vilib>:"NT Write Value.vi"("Boolean"=FALSE, "Name"="CW Deploy") -> ()  [unwired: 9 in, 1 out]
            }
          }
        }
      }
      n267 = call-poly <vilib>:"NT Write Value.vi"("Boolean"=w427, "Name"="Lift Lock") -> ()  [unwired: 9 in, 1 out]
    }
  }
  n268 = disable-structure shown="Disabled" {
    frame Disabled {
      n269 = case shown="True" w474 {
        frame False {
        }
        frame True {
          n270 = call-poly <vilib>:"NT Write Value.vi"("String"="Red", "Name"="Color Wheel") -> ()  [unwired: 9 in, 1 out]
        }
      }
      n271 = case shown="True" w477 {
        frame False {
        }
        frame True {
          n272 = call-poly <vilib>:"NT Write Value.vi"("String"="Yellow", "Name"="Color Wheel") -> ()  [unwired: 9 in, 1 out]
        }
      }
      n273 = case shown="True" w476 {
        frame False {
        }
        frame True {
          n274 = call-poly <vilib>:"NT Write Value.vi"("String"="Rotation", "Name"="Color Wheel") -> ()  [unwired: 9 in, 1 out]
        }
      }
      n275 = case shown="True" w471 {
        frame False {
        }
        frame True {
          n276 = call-poly <vilib>:"NT Write Value.vi"("String"="Green", "Name"="Color Wheel") -> ()  [unwired: 9 in, 1 out]
        }
      }
      n277 = case shown="True" w470 {
        frame False {
        }
        frame True {
          n278 = call-poly <vilib>:"NT Write Value.vi"("String"="Blue", "Name"="Color Wheel") -> ()  [unwired: 9 in, 1 out]
        }
      }
      n279 = Compound Arithmetic op=XOR(w477, w476, w471, w470) -> (w473:bool, w475:bool)
      n280 = Not(x=w473) -> (.not. x?=w472:bool)
      n281 = case shown="True" w472 {
        frame False {
        }
        frame True {
          n282 = call-poly <vilib>:"NT Write Value.vi"("String"="Off", "Name"="Color Wheel") -> ()  [unwired: 9 in, 1 out]
        }
      }
    }
    frame Enabled {
    }
  }
